vi "MQTT_Read_Published_Message.vi"(8 "error in (no error)":errorcluster, 9 "timeout ms (25000)":i32=25000, 11 "connection ID":refnum<k5>) -> (0 "error out":errorcluster, 1 "Message":string="MQIsdp", 2 "Topic Name":string="Topic", 3 "connection ID out":refnum<k5>, 4 "MessageType":T1, 5 "Message ID":u16=1 format="%x")   [LabVIEW 2018, in "MQTT_Functions.lvlib"]
uses:
  MQTT_Functions.lvlib
  Controls/MessageType.ctl
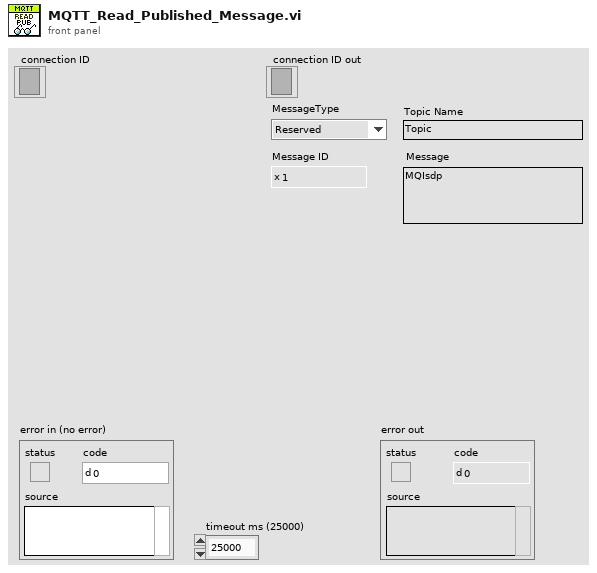
[diagram p1: front panel]
types:
  T1 = typedef "MQTT_Functions.lvlib/MessageType.ctl" = enum32{"Reserved", "CONNECT", "CONNACK", "PUBLISH", "PUBACK", "PUBREC", "PUBREL", "PUBCOMP", "SUBSCRIBE", "SUBACK", "UNSUBSCRIBE", "UNSUBACK", "PINGREQ", "PINGRESP", "DISCONNECT", "Reserved2"}
  T2 = typedef "MQTT_Functions.lvlib/QoS.ctl" = enum8{"At most once", "At least once", "Exactly once", "Reserved"}
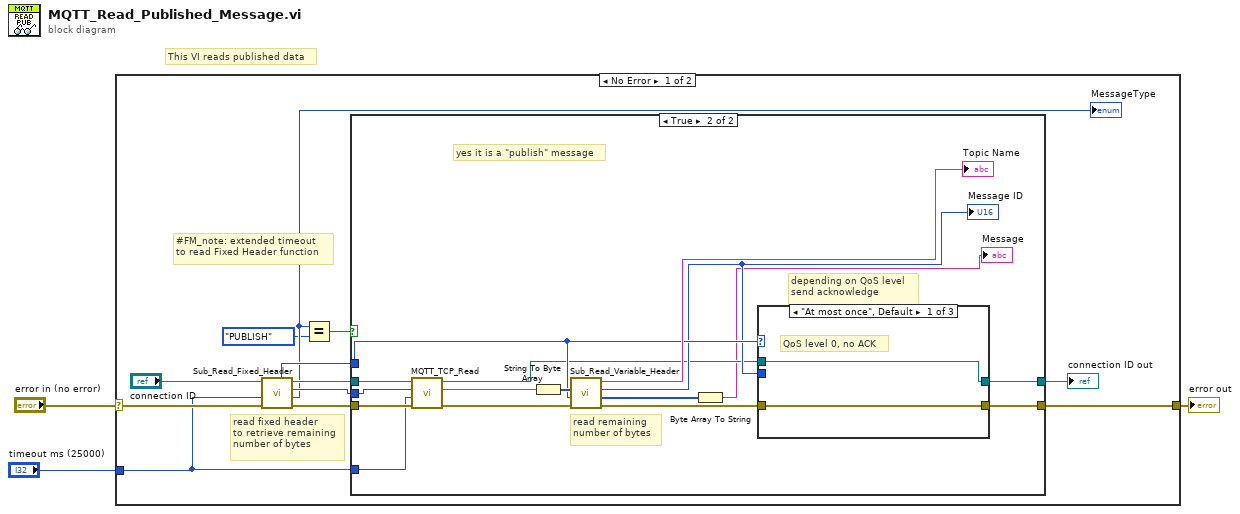
[diagram p0: block diagram]
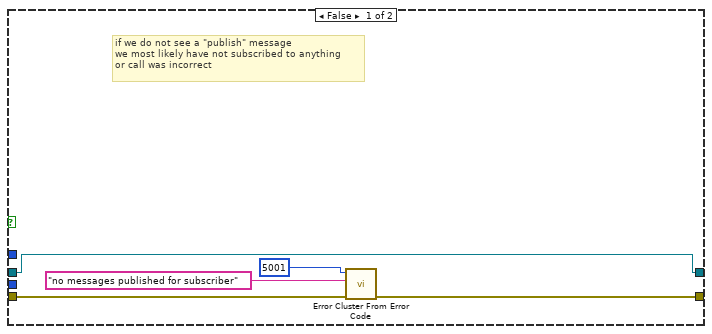
[diagram p2: hidden frame]
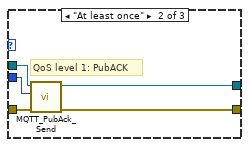
[diagram p3: hidden frame]
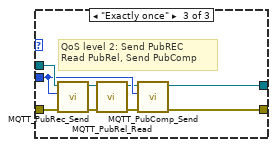
[diagram p4: hidden frame]
diagram:
  # "This VI reads published data"
  n1 = case shown="No Error" "error in (no error)" {
    selector: "error in (no error)" -> [w14 w53]
    tunnel: [w8 w53] -> w2
    tunnel: "timeout ms (25000)" -> [w4 _]
    frame No Error {
      # "#FM_note: extended timeout\nto read Fixed Header function"
      # "read fixed header \nto retrieve remaining\nnumber of bytes"
      n2 = call "Sub_Read_Fixed_Header.vi"("error in (no error)"=w14, "timeout ms (25000)"=w4, "connection ID"="connection ID") -> ("error out"=w11:errorcluster, "MessageType"=w7:T1, "Remaining Length"=w13:u32, "connection ID out"=w12:refnum<k5>, "QoS Level"=w10:T2)  [unwired: 2 in, 2 out]
      "MessageType" <- w7
      n3 = Equal?(x=w7, y=MessageType."PUBLISH") -> (x = y?=w5:bool)
      n4 = case shown="True" w5 {
        tunnel: w13 -> [_ w35]
        tunnel: w12 -> [w16 w34]
        tunnel: w11 -> [w20 w33]
        tunnel: w10 -> [_ w29]
        tunnel: [w16 w26] -> w9
        tunnel: [w17 w25] -> w8
        tunnel: w4 -> [_ w21]
        frame False {
          # "if we do not see a \"publish\" message\nwe most likely have not subscribed to anything\nor call was incorrect"
          n5 = call <vilib>:"Error Cluster From Error Code.vi"("error in (no error)"=w20, "error message (\"\")"="no messages published for subscriber" ("error message (\"\")"), "error code (0)"=5001) -> ("error out"=w17:errorcluster)  [unwired: 6 in]
        }
        frame True {
          # "yes it is a \"publish\" message"
          # "depending on QoS level\nsend acknowledge"
          # "read remaining\nnumber of bytes"
          n6 = call "MQTT_TCP_Read.vi"("error in (no error)"=w33, "timeout ms (25000)"=w21, "bytes to read"=w35, "connection ID"=w34) -> ("error out"=w30:errorcluster, "data out"=w32:string, "connection ID out"=w27:refnum<k5>)  [unwired: 5 in]
          n7 = String To Byte Array(string=w32) -> (unsigned byte array=w31:u8[])
          n8 = call "Sub_Read_Variable_Header.vi"("error in (no error)"=w30, "QoS"=w29, "Variable Header"=w31) -> ("error out"=w24:errorcluster, "remaining bytes"=w22:u8[], "Message ID"=w28:u16, "Topic Name"=→"Topic Name":string)  [unwired: 5 in]
          "Message ID" <- w28
          n9 = Byte Array To String(unsigned byte array=w22) -> (string=→"Message":string)
          n10 = case shown="\"At most once\", Default" w29 {
            tunnel: w28 -> [_ w43 w48]
            tunnel: w24 -> [w37 w42 w52]
            tunnel: w27 -> [w38 w41 w51]
            tunnel: [w38 w40 w50] -> w26
            tunnel: [w37 w39 w49] -> w25
            frame "At most once", Default {
              # "QoS level 0, no ACK"
            }
            frame "At least once" {
              # "QoS level 1: PubACK"
              n11 = call "MQTT_PubAck_Send.vi"("error in (no error)"=w42, "Message ID"=w43, "connection ID"=w41) -> ("error out"=w39:errorcluster, "connection ID out"=w40:refnum<k5>)  [unwired: 6 in, 1 out]
            }
            frame "Exactly once" {
              # "QoS level 2: Send PubREC\nRead PubRel, Send PubComp"
              n12 = call "MQTT_PubRec_Send.vi"("error in (no error)"=w52, "Message ID"=w48, "connection ID"=w51) -> ("error out"=w45:errorcluster, "connection ID out"=w44:refnum<k5>)  [unwired: 6 in, 1 out]
              n13 = call "MQTT_PubRel_Read.vi"("error in (no error)"=w45, "connection ID"=w44) -> ("error out"=w46:errorcluster, "connection ID out"=w47:refnum<k5>)  [unwired: 7 in, 1 out]
              n14 = call "MQTT_PubComp_Send.vi"("error in (no error)"=w46, "Message ID"=w48, "connection ID"=w47) -> ("error out"=w49:errorcluster, "connection ID out"=w50:refnum<k5>)  [unwired: 6 in, 1 out]
            }
          }
        }
      }
      "connection ID out" <- w9
    }
    frame Error {
    }
  }
  "error out" <- w2
